vi "Remote_Sense_Test_v1.vi"(10 "HMP VISA":refnum<visa-resource-name>, 11 "ControlBoard VISA":refnum<visa-resource-name>="ControlBoard") -> (2 "Control Board OUT":refnum<visa-resource-name>, 3 "Pass?":bool)   [LabVIEW 2019]
uses:
  Ctls/Powersupply_Auto_Enum_v1.ctl
panel:
  out "Message OUT":string
  out "MSE Array":dbl[](array[numeric])
  out "Voltage Readings":dbl[][](array[numeric])
  in  "Message IN":string
  out "error out":errorcluster
  in  "error in (no error)":errorcluster
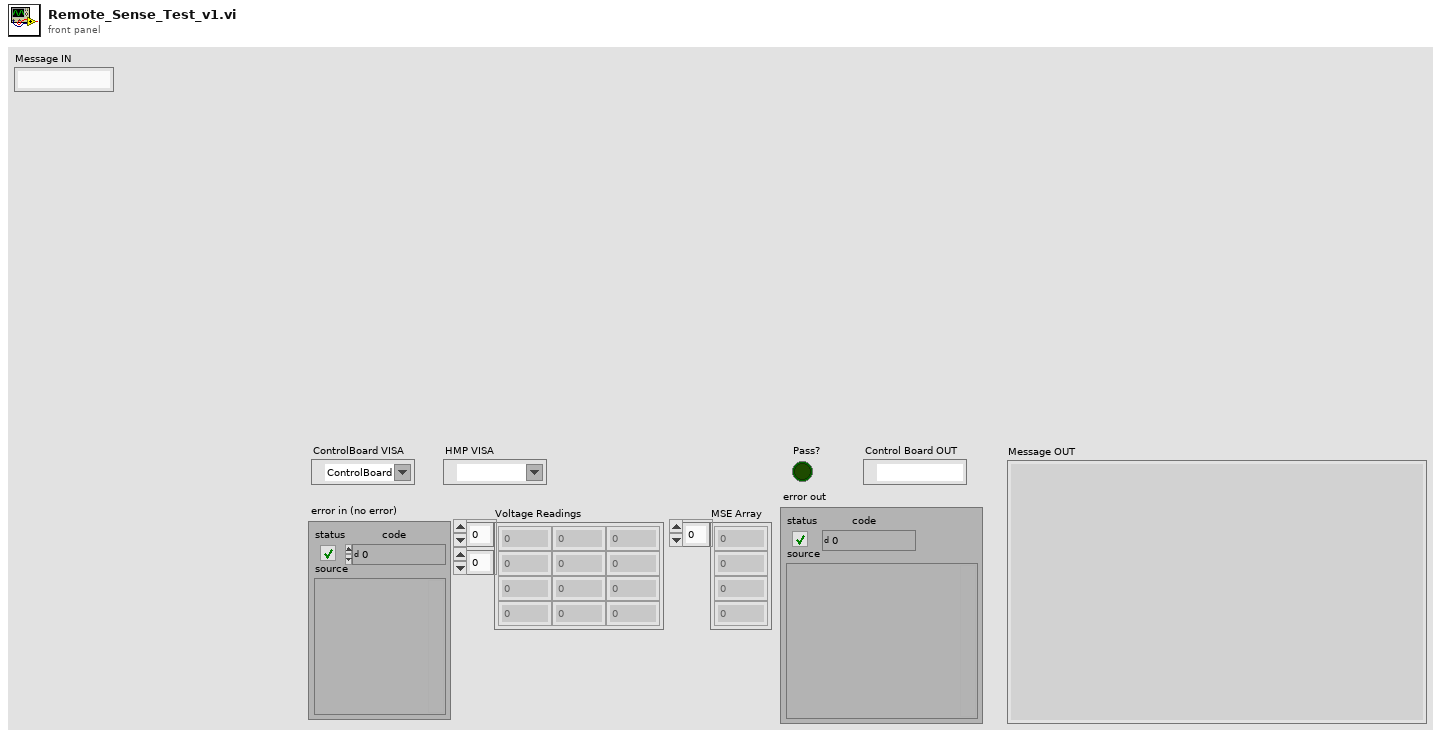
[diagram p1: front panel]
types:
  T1 = typedef "Powersupply_Auto_Enum_v1.ctl" = enum16{"Off", "Control Power", "HMP2020 Control + DC32V", "HMP2020 Control + DC8V", "HMP4040 Control + DC32V", "HMP4040 Control +DC8V"}
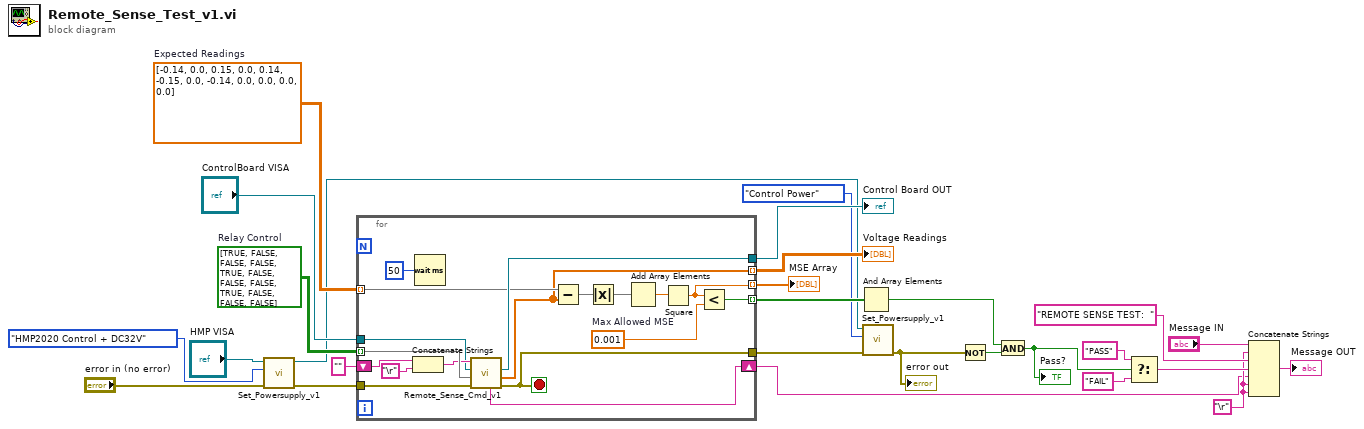
[diagram p0: block diagram]
diagram:
  w9 = dbl[][] [[-0.14, 0.0, 0.15], [0.0, 0.14, -0.15], [0.0, -0.14, 0.0], [0.0, 0.0, 0.0]]  # Expected Readings
  w15 = "\r"
  w25 = bool[][] [[TRUE, FALSE, FALSE], [FALSE, TRUE, FALSE], [FALSE, FALSE, TRUE], [FALSE, FALSE, FALSE]]  # Relay Control
  n1 = call "Set_Powersupply_v1.vi"("error in (no error)"="error in (no error)", "Enum"=Powersupply_Auto_Enum_v1."HMP2020 Control + DC32V", "HMP VISA"="HMP VISA") -> ("error out"=w5:errorcluster, "HMP VISA Out"=w2:refnum<visa-resource-name>)  [unwired: 7 in]
  n2 = for {
    tunnel: [w43] -> w4
    tunnel: [w45] -> w27
    tunnel: w5 -> [w44]
    tunnel: w9 -> [w40] mode=indexing
    tunnel: [w37] -> w26 mode=indexing
    tunnel: w25 -> [w36] mode=indexing
    tunnel: [w35] -> w22 mode=indexing
    tunnel: [w34] -> w21 mode=indexing
    shift-right: [w28] -> w13
    shift-left: "" -> [w33]
    tunnel: "ControlBoard VISA" -> [w29]
    stop <- w43 stop-if-true
    w38 = 0.001  # Max Allowed MSE
    n3 = Concatenate Strings(w33, "\r") -> (w32:string)
    n4 = Wait (ms)(milliseconds to wait=u32 50) -> ()  [unwired: 1 out]
    n5 = call "Remote_Sense_Cmd_v1.vi"("error in (no error)"=w44, "Relay Control"=w36, "ControlBoard VISA"=w29, "RemoteSenseRelayTask"=w32) -> ("error out"=w43:errorcluster, "Voltage Array"=w35:dbl[], "Control Board OUT"=w45:refnum<visa-resource-name>, "Message OUT"=w28:string)  [unwired: 3 in, 1 out]
    n6 = Subtract(x=w40, y=w35) -> (x-y=w42:dbl[])
    n7 = Absolute Value(x=w42) -> (abs(x)=w41:dbl[])
    n8 = Add Array Elements(numeric array=w41) -> (sum=w39:dbl)
    n9 = Square(x=w39) -> (x^2=w34:dbl)
    n10 = Less?(x=w34, y=w38) -> (x < y?=w37:bool)
  }
  "Voltage Readings" <- w22
  "MSE Array" <- w21
  "Control Board OUT" <- w27
  n11 = And Array Elements(Boolean array=w26) -> (logical AND=w24:bool)
  n12 = call "Set_Powersupply_v1.vi"("error in (no error)"=w4, "Enum"=Powersupply_Auto_Enum_v1."Control Power", "HMP VISA"=w2) -> ("error out"=w3:errorcluster)  [unwired: 7 in, 1 out]
  "error out" <- w3
  n13 = Not(x=w3) -> (.not. x?=w23:bool)
  n14 = And(x=w24, y=w23) -> (x .and. y?=w14:bool)
  "Pass?" <- w14
  n15 = Select(t="PASS", s=w14, f="FAIL") -> (s? t:f=w19:string)
  n16 = Concatenate Strings("Message IN", w15, "REMOTE SENSE TEST:  ", w19, w13, w15, w15) -> (→"Message OUT":string)
